vi "Test.vi"() -> ()   [LabVIEW 2014]
uses:
  <vilib>/addons/Modulation/Digital/General/MT Generate Bits (Galois, PN Order).vi
  <vilib>/addons/Modulation/Analog/support/mod_Set Error Source.vi
  <vilib>/addons/Modulation/Digital/Support/Common/Validators/mod_Generate Bits Validate.vi
  <vilib>/addons/Modulation/Digital/General/MT Generate PSK System Parameters(M).vi
  <vilib>/addons/Modulation/Digital/Support/Common/Validators/mod_Generate Filter Coefficients Validate.vi
  <vilib>/addons/Modulation/Digital/General/subVIs/mod_Generate Filter Coefficients.vi
  <vilib>/addons/Modulation/Digital/General/subVIs/mod_Generate Bits PN Sequence.vi
  <vilib>/addons/Modulation/niDMT.lvlib
panel:
  out "output bit stream":i8[](array[numeric])
  out "appended array":i8[](array[numeric])
  out "Number of Packets":i32
  out "File Length (bits)":i32
  in  "PN sequence order\nfor Sync Bits":i32=31 caption="PN sequence order (9)"
  in  "Packet Pad \n[samples]":i32=200
  in  "Packet Parameters":T1={"Guard Bits "=30, "Sync Bits"=20, "Message Bits"=128}
  in  "synchronization parameters":T2={"expected sync location (symbols)"=-1, "sync sequence"=[], "sync location uncertainty (symbols)"=0, "sync indent (symbols)"=0} {"sync sequence" format="%.2f"}
  in  "filter parameters":T3={"Alpha"=0.5, "Filter Length"=6, "TX Filter"=enum."Root Raised Cos"} {"Alpha" format="%.2f"}
  out "Symbol Rate":dbl
  out "Padding Bits":i32
  in  "Tx IQ Sampling\nRate [s/sec]":dbl
  in  "modulation type":T4(ring)
  out "bits per symbol":i32
  in  "differential PSK":enum16{"disable", "enable"}(ring)
  in  "M-PSK (4)":i32=4
  in  "samples per symbol (16)":i32=16
  in  "PSK type":u16(ring) items=["normal", "shifted", "offset"]
  in  "Input file":path
  in  "file path (use dialog)":path
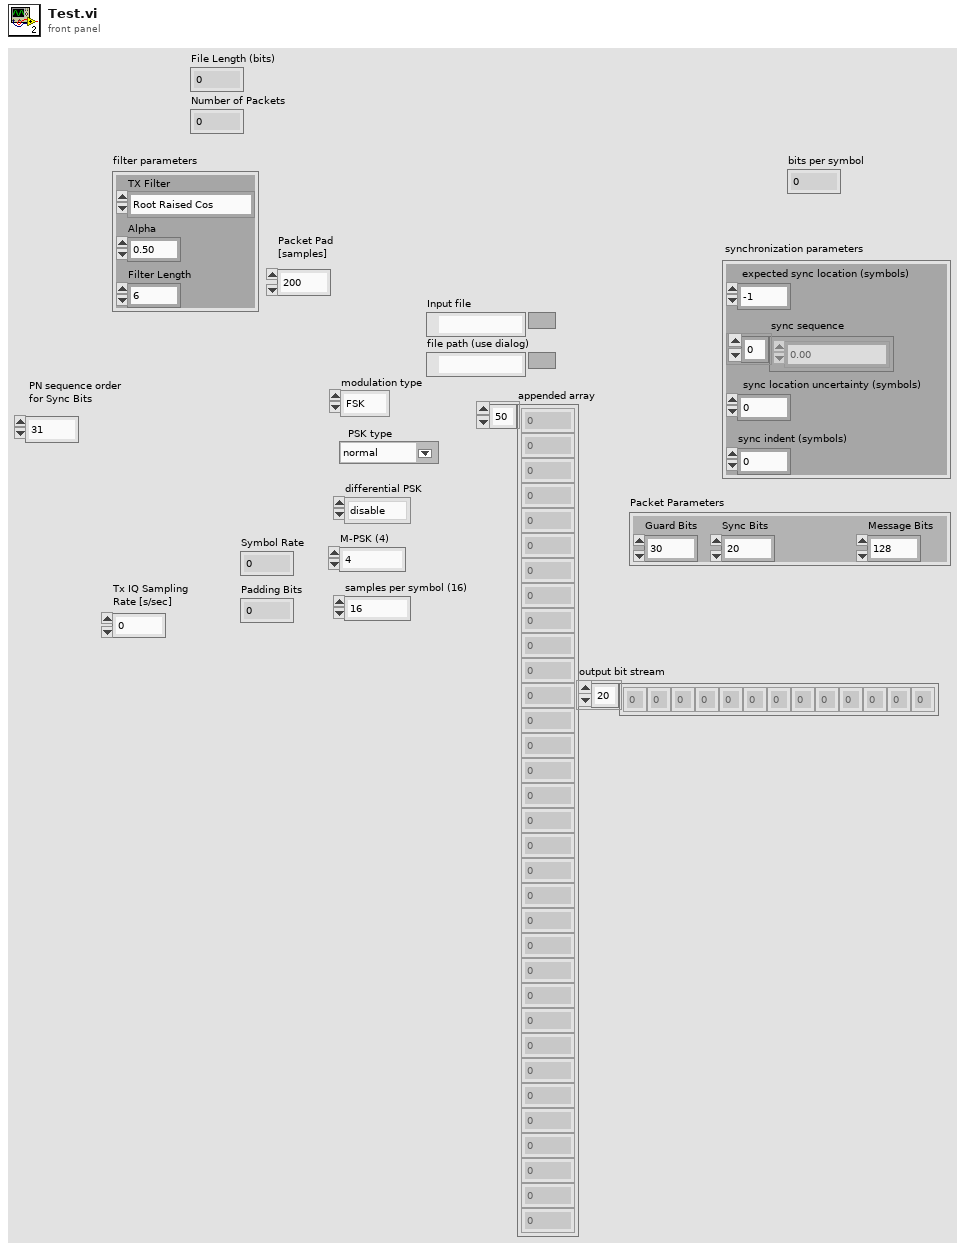
[diagram p1: front panel]
types:
  T1 = cluster{"Guard Bits ":i32, "Sync Bits":i32, "Message Bits":i32}
  T2 = cluster{"expected sync location (symbols)":i32, "sync sequence":cdb[], "sync location uncertainty (symbols)":i32, "sync indent (symbols)":i32}
  T3 = cluster{"Alpha":dbl, "Filter Length":i32, "TX Filter":enum16{"none", "Raised Cosine", "Root Raised Cos", "Gaussian"}}
  T4 = enum16{"FSK", "PSK", "QAM", "MSK", "PAM", "ASK", "CPM"}
  T5 = cluster{"samples per symbol (16)":i32, "symbol map":cdb[], "differential PSK":enum16{"disable", "enable"}, "PSK type":u16}
  T6 = enum16{"none", "Raised Cosine", "Root Raised Cos", "Gaussian"}
  T7 = typedef "niAMT.lvlib/Complex Data Waveform.ctl" = cluster{"t0":dbl, "dt":dbl, "Y":cdb[]}
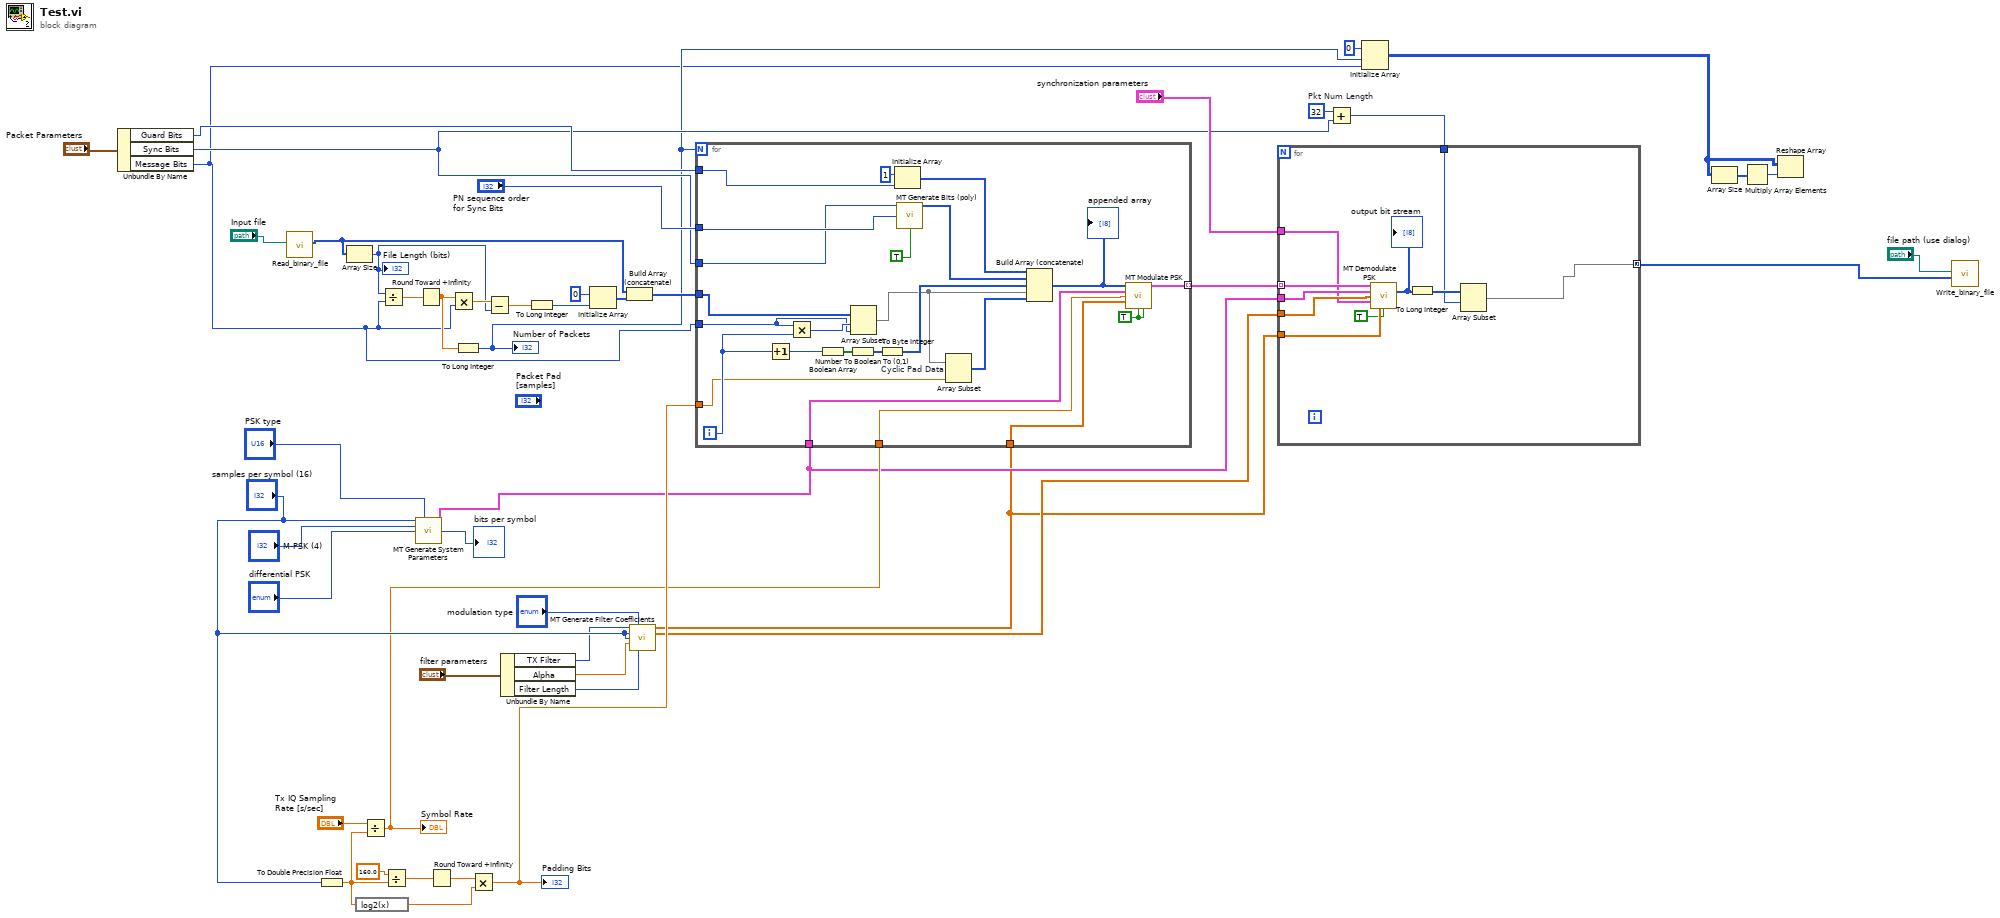
[diagram p0: block diagram]
diagram:
  w10 = 32  # Pkt Num Length
  n1 = Unbundle By Name("Packet Parameters") -> ("Guard Bits"=w17:i32, "Sync Bits"=w9:i32, "Message Bits"=w5:i32)
  n2 = call "Read_binary_file.vi"("Open path"="Input file") -> ("message bitstream"=w22:i8[])  [unwired: 10 in]
  n3 = To Double Precision Float(number="samples per symbol (16)") -> (double precision float=w40:dbl)
  n4 = Array Size(array=w22) -> (size(s)=w27:i32)
  "File Length (bits)" <- w27
  n5 = expression code="log2(x)"(w40) -> (w39:dbl)
  n6 = Divide(x="Tx IQ Sampling\nRate [s/sec]", y=w40) -> (x/y=w16:dbl)
  "Symbol Rate" <- w16
  n7 = Divide(x=w27, y=w5) -> (x/y=w29:dbl)
  n8 = Divide(x=160.0, y=w40) -> (x/y=w37:dbl)
  n9 = call-poly <vilib>:"MT Generate System Parameters.vi"("samples per symbol (16)"="samples per symbol (16)", "PSK type"="PSK type", "M-PSK (4)"="M-PSK (4)", "differential PSK"="differential PSK") -> ("PSK system parameters"=w14:T5, "bits per symbol"=→"bits per symbol":i32)  [unwired: 9 in, 1 out]
  n10 = Round Toward +Infinity(x=w29) -> (ceil(x): smallest int >= x=w25:dbl)
  n11 = Round Toward +Infinity(x=w37) -> (ceil(x): smallest int >= x=w38:dbl)
  n12 = Multiply(x=w25, y=w5) -> (x*y=w28:dbl)
  n13 = To Long Integer(number=w25) -> (32bit integer=w6:i32)
  "Number of Packets" <- w6
  n14 = Multiply(x=w38, y=w39) -> (x*y=w21:dbl)
  "Padding Bits" <- w21
  n15 = Subtract(x=w28, y=w27) -> (x-y=w26:dbl)
  n16 = Unbundle By Name("filter parameters") -> ("TX Filter"=w33:T6, "Alpha"=w32:dbl, "Filter Length"=w31:i32)
  n17 = To Long Integer(number=w26) -> (32bit integer=w24:i32)
  n18 = Initialize Array(i8 0 ("element"), w24) -> (w23:i8[])
  n19 = Build Array (concatenate)(w22, w23) -> (w20:i8[])
  n20 = call <vilib>:"MT Generate Filter Coefficients.vi"("pulse shaping filter (none)"=w33, "modulation type"="modulation type", "pulse shaping samples per symbol (16)"="samples per symbol (16)", "matched samples per symbol (16)"="samples per symbol (16)", "filter parameter"=w32, "filter length (symbols)"=w31) -> ("pulse shaping filter coefficients"=w11:dbl[], "matched filter coefficients"=w13:dbl[])  [unwired: 7 in, 1 out]
  n21 = for {
    N: w6 -> [_]
    tunnel: w21 -> [w57]
    tunnel: w20 -> [w71]
    tunnel: w5 -> [w70]
    tunnel: "PN sequence order\nfor Sync Bits" -> [w67]
    tunnel: w17 -> [w66]
    tunnel: w9 -> [w65]
    tunnel: w14 -> [w52]
    tunnel: w16 -> [w51]
    tunnel: w11 -> [w50]
    tunnel: [w49] -> w15 mode=indexing
    i -> [w59]
    w54 = TRUE ("reset? (T)")
    n22 = Increment(x=w59) -> (x+1=w60:i32)
    n23 = Multiply(x=w70, y=w59) -> (x*y=w72:i32)
    n24 = Number To Boolean Array(number=w60) -> (Boolean array=w61:bool[])
    n25 = Boolean To (0,1)(Boolean=w61) -> (0, 1=w62:i16[])
    n26 = Array Subset(array=w71, index=w72, length=w70) -> (w56:i8[])
    n27 = To Byte Integer(number=w62) -> (8bit integer=w58:i8[])
    n28 = Initialize Array(i8 1 ("Numeric"), w66) -> (w64:i8[])
    n29 = call-poly <vilib>:"MT Generate Bits (poly).vi"("total bits (128)"=w65, "PN sequence order (9)"=w67, "reset? (T)"=TRUE ("Reset? (T)")) -> ("output bit stream"=w63:i8[])  [unwired: 10 in, 2 out]
    n30 = Array Subset "Cyclic Pad Data"(array=w56, length=w57) -> (w55:i8[])  [unwired: 1 in]
    n31 = Build Array (concatenate)(w64, w63, w58, w56, w55) -> (w53:i8[])
    "appended array" <- w53
    n32 = call <vilib>:"MT Modulate PSK.vi"("input bit stream"=w53, "PSK system parameters"=w52, "symbol rate (Hz)"=w51, "pulse shaping filter coefficients"=w50, "reset? (T)"=w54, "flush buffers? (F)"=w54) -> ("output complex waveform"=w49:T7)  [unwired: 7 in, 2 out]
  }
  n33 = Add(x=w10, y=w9) -> (x+y=w8:i32)
  n34 = for {
    tunnel: w15 -> [w82] mode=indexing
    tunnel: w14 -> [w81]
    tunnel: w13 -> [w80]
    tunnel: "synchronization parameters" -> [w79]
    tunnel: w11 -> [w78]
    tunnel: w8 -> [w74]
    tunnel: [w73] -> w1 mode=concatenating
    n35 = call <vilib>:"MT Demodulate PSK.vi"("input complex waveform"=w82, "PSK system parameters"=w81, "matched filter coefficients"=w80, "synchronization parameters"=w79, "pulse shaping filter coefficients"=w78, "reset? (T)"=TRUE) -> ("output bit stream"=w75:i8[])  [unwired: 5 in, 4 out]
    "output bit stream" <- w75
    n36 = To Long Integer(number=w75) -> (32bit integer=w76:i32[])
    n37 = Array Subset(array=w76, index=w74) -> (w73:i32[])  [unwired: 1 in]
  }
  n38 = Initialize Array(0, w6, w5) -> (w2:i32[][])
  n39 = Array Size(array=w2) -> (size(s)=w3:i32[])
  n40 = Multiply Array Elements(1:w3) -> (0:w4:i32)
  n41 = Reshape Array(w2, w4) -> ()  [unwired: 1 out]
  n42 = call "Write_binary_file.vi"("output bit stream 3"=w1, "Save path"="file path (use dialog)") -> ()  [unwired: 10 in]
